vi "Gazebo_SetLink_Init.vi"(11 "Definitions":T2={"Topic"="/gazebo/set_link_state", "Type"="gazebo_msgs/LinkState", "Action"=enum."Publisher", "Update (ms)"=1, "write queue"=1}) -> (3 "ROS out":T3)   [LabVIEW 2012]
doc: "Initializes the ROS topic /gazebo/set_link_states .\n\nThe input does not need to be wired and is included only for debugging purposes."
uses:
  <userlib>/rosforlv/ROS/Code/SubVIs/_ROSControl.ctl
  <userlib>/rosforlv/ROS/Code/SubVIs/_ROSDirection.ctl
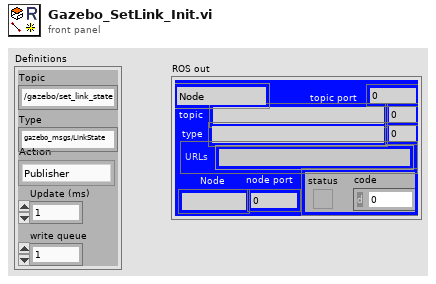
[diagram p1: front panel]
types:
  T1 = typedef "_ROSDirection.ctl" = enum16{"Node", "Publisher", "Subscriber", "Service Client"}
  T2 = cluster{"Topic":string, "Type":string, "Action":T1, "Update (ms)":u16, "write queue":u16}
  T3 = typedef "_ROSControl.ctl" = cluster{"topic port":u16, "Node":string, "topic":string, "type":string, "node port":u32, "error ":errorcluster, "Direction":T1, "APIs":string[], "Update (ms)":u16, "write queue":u16}
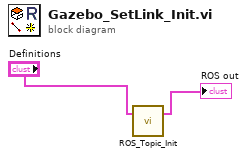
[diagram p0: block diagram]
diagram:
  n1 = call <userlib>:"ROS_Topic_Init.vi"("Definitions"="Definitions") -> ("ROS out"=→"ROS out":T3)  [unwired: 2 in]
